vi "习5.6.vi"() -> ()   [LabVIEW 2017]
uses:
  <vilib>/measure/NI_MABase.lvlib
panel:
  out "最大值":dbl
  out "大小":i32
  out "Y":dbl[](array[numeric])
  out "dt":dbl
  out "signal out":waveform(dbl) caption="信号输出"
  in  "频率":dbl=10.0 format="%0.2p"
  in  "幅值":dbl=1.0 format="%0.2p"
  in  "相位":dbl format="%.2p"
  in  "采样信息":cluster{"Fs":dbl, "#s":dbl}={"Fs"=1000.0, "#s"=1000.0} {"Fs" format="%.2p"}
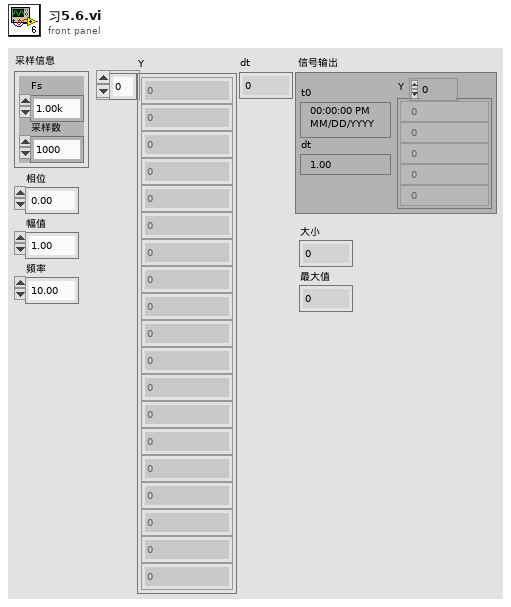
[diagram p1: front panel]
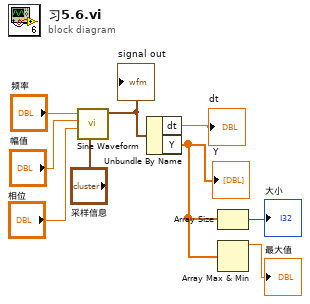
[diagram p0: block diagram]
diagram:
  n1 = call <vilib>:"Sine Waveform.vi"("sampling info"="采样信息", "phase"="相位", "amplitude"="幅值", "frequency"="频率") -> ("signal out"=w5:waveform(dbl))  [unwired: 6 in, 1 out]
  "signal out" <- w5
  n2 = Unbundle By Name(w5) -> ("dt"=→"dt":dbl, "Y"=w2:dbl[])
  "Y" <- w2
  n3 = Array Size(array=w2) -> (size(s)=→"大小":i32)
  n4 = Array Max & Min(array=w2) -> (max value=→"最大值":dbl)  [unwired: 3 out]
